vi "EE_SetMarker.vi"(8 "error in (no error)":errorcluster, 10 "Marker Value":i32, 11 "EmotivEpocHeadsetControls in":refnum<class "EmotivEpocHeadsetControls.lvclass">) -> (0 "error out":errorcluster, 3 "EmotivEpocHeadsetControls out":refnum<class "EmotivEpocHeadsetControls.lvclass">)   [LabVIEW 2016, in "Emotiv Epoc.lvlib" / "EmotivEpocHeadsetControls.lvclass"]
uses:
  EmotivEpocHeadsetControls.lvclass
  EmotivEpocHeadsetControls.lvclass/EmotivEpocHeadsetControls.ctl
panel:
  # "This VI is a part of BCI Design library, http://www.ru-bci.org \nCopyright © 2020, Sotnikov Peter, All rights reserved. License: CC BY-NC 4.0"
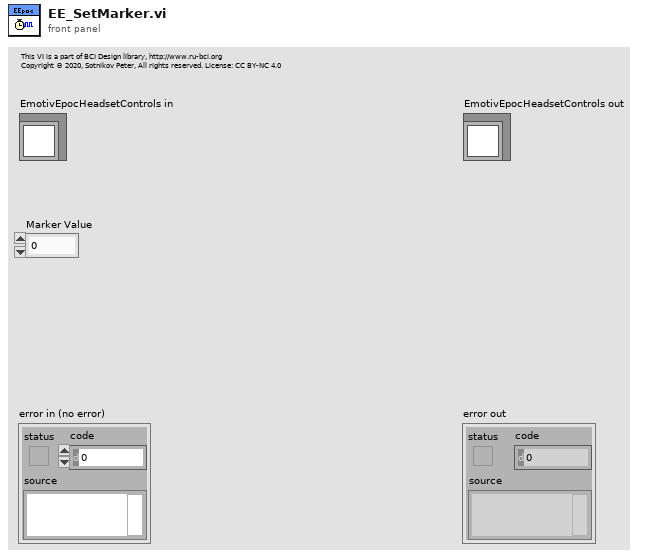
[diagram p1: front panel]
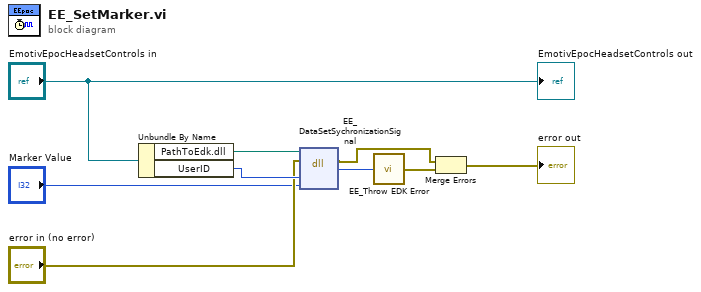
[diagram p0: block diagram]
diagram:
  n1 = Unbundle By Name("EmotivEpocHeadsetControls in") -> ("PathToEdk.dll"=w8:path, "UserID"=w7:u32)
  n2 = dll-call lib="C:/Program Files/Emotiv Development Kit_v1.0.0.3-PREMIUM/edk.dll" fn="EE_DataSetSychronizationSignal"(path in=w8, error in="error in (no error)", "userId"=w7, "marker"="Marker Value") -> (error out=w2:errorcluster, "EDK_ERROR_CODE"=w4:i32)  [unwired: 3 in, 1 out]
  n3 = call "EE_Throw EDK Error.vi"("edkErrorCode"=w4) -> ("edkErroCode"=w3:errorcluster)
  n4 = Merge Errors(w2, w3) -> (→"error out":errorcluster)
  "EmotivEpocHeadsetControls out" <- "EmotivEpocHeadsetControls in"
